vi "verify_controlLaw.vi"() -> ()   [LabVIEW 2014]
uses:
  controls/Xdelay.ctl
panel:
  out "u(k) (saturated)":sgl
  out "x^(k+1) = Ax + Bu + Lye":sgl[](array[numeric])
  out "Xd_out(k+1)":T1 caption="Xd_out"
  in  "Xd_in":T1=[0.0, 0.0, 0.0, 0.0, 0.0, 0.0, 0.0, 0.0, 0.0, 0.0, 0.0, 0.0]
  in  "x^(k)":sgl[](array[numeric])=[0.0, 0.0, 0.0, 0.0, 0.0, 0.0, 0.0, 0.0, 0.0, 0.0, 0.0, 0.0, 0.0, 0.0, 0.0, 0.0, 0.0, 0.0, 0.0, 0.0, 0.0, 0.0, 0.0, 0.0, 0.0]
  in  "Cluster":T2={"umax"=3.0, "y_ref(k)"=0.0, "Ki"=0.0, "y(k) (from plant)"=0.0, "ND"=0, "NS"=0, "u_Kx_ref(k)"=0.0} {"u_Kx_ref(k)" format="%#_13g"; "Ki" format="%#_13g"; "y_ref(k)" format="%#_13g"; "umax" format="%#_13g"}
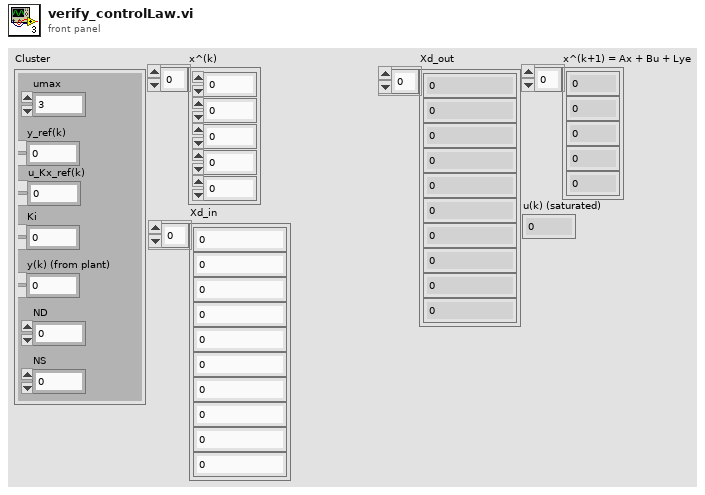
[diagram p1: front panel]
types:
  T1 = typedef "Xdelay.ctl" = sgl[]
  T2 = cluster{"umax":sgl, "y_ref(k)":sgl, "Ki":sgl, "y(k) (from plant)":sgl, "ND":i16, "NS":i16, "u_Kx_ref(k)":sgl}
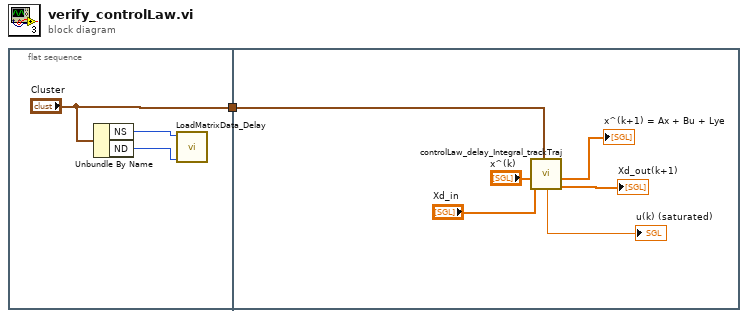
[diagram p0: block diagram]
diagram:
  n1 = flat-sequence {
    tunnel: ["Cluster"] -> w1
    tunnel: w1 -> [w5]
    frame #0 {
      n2 = Unbundle By Name("Cluster") -> ("NS"=w3:i16, "ND"=w2:i16)
      n3 = call "LoadMatrixData_Delay.vi"("Nd"=w2, "NS"=w3) -> ()  [unwired: 9 in, 1 out]
    }
    frame #1 {
      n4 = call "controlLaw_delay_Integral_trackTraj.vi"("Cluster"=w5, "Xd_in"="Xd_in", "x^(k)"="x^(k)") -> ("Xd_out(k+1)"=→"Xd_out(k+1)":T1, "x^(k+1) = Ax + Bu + Lye"=→"x^(k+1) = Ax + Bu + Lye":sgl[], "u(k) (saturated)"=→"u(k) (saturated)":sgl)  [unwired: 6 in]
    }
  }
